vi "Teleop.vi"(10 "Match Info":T1={"Autonomous Elapsed Seconds"=0.0, "TeleOp Elapsed Seconds"=0.0, "Disabled Elapsed Seconds"=0.0, "Visited Autonomous"=FALSE, "Visited TeleOp"=FALSE, "Visited Disabled"=FALSE, "Autonomous Settings"={"Autonomous Style"=enum."Independent", "VI Refnum"=refnum}}, 11 "Call Context":T2) -> ()   [LabVIEW 2014]
doc: "This VI is called for each TeleOp packet received from the DS where the robot is not disabled. It is often used to read from the joysticks and update I/O or to update setpoints for timed control loops. It should complete and return within 20 milliseconds or it may miss DS packets."
uses:
  <vilib>/Rock Robotics/WPI/DriverStation/WPI_DriverStationDerivedRobotMode.ctl
  <vilib>/Rock Robotics/WPI/DriverStation/WPI_DriverStationMatch Info.ctl
  Robot Global Data.vi
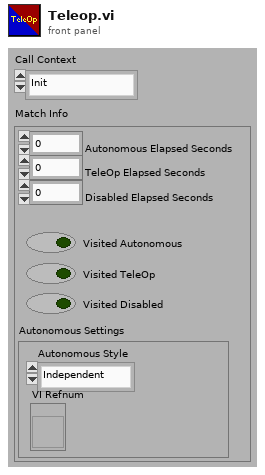
[diagram p1: front panel]
types:
  T1 = typedef "WPI_DriverStationMatch Info.ctl" = cluster{"Autonomous Elapsed Seconds":dbl, "TeleOp Elapsed Seconds":dbl, "Disabled Elapsed Seconds":dbl, "Visited Autonomous":bool, "Visited TeleOp":bool, "Visited Disabled":bool, "Autonomous Settings":cluster{"Autonomous Style":enum16{"Iterative", "Independent"}, "VI Refnum":refnum<vi>}}
  T2 = typedef "WPI_DriverStationDerivedRobotMode.ctl" = enum16{"Init", "Execute", "Stop"}
  T3 = cluster{"axis 3 (throttle)":dbl, "axis 1 (x)":dbl, "axis 2 (y)":dbl}
  T4 = cluster{"Trigger":bool, "Top 1":bool, "Side Trigger":bool, "Top 2":bool, "Top 3":bool, "Top 4":bool, "Bottom 1":bool, "Bottom 2":bool, "Bottom 3":bool, "Bottom 4":bool, "Bottom 5":bool, "Bottom 6":bool}
  T5 = cluster{"axis 1 (x)":dbl, "axis 2 (y)":dbl, "axis 3 (throttle)":dbl, "axis 4":dbl, "axis 5":dbl, "axis 6":dbl}
  T6 = typedef "WPI_AnalogChannelDevRef.ctl" = cluster{"DevStatus":errorcluster, "Analog Module":T7, "Analog Channel":T8}
  T7 = typedef "FPGA_TypedefAnalogModule.ctl" = enum16{"Analog Module 1", "Analog Module 2"}
  T8 = typedef "FPGA_AIChannel.ctl" = enum8{"AI 1", "AI 2", "AI 3", "AI 4", "AI 5", "AI 6", "AI 7", "AI 8", "Invalid"}
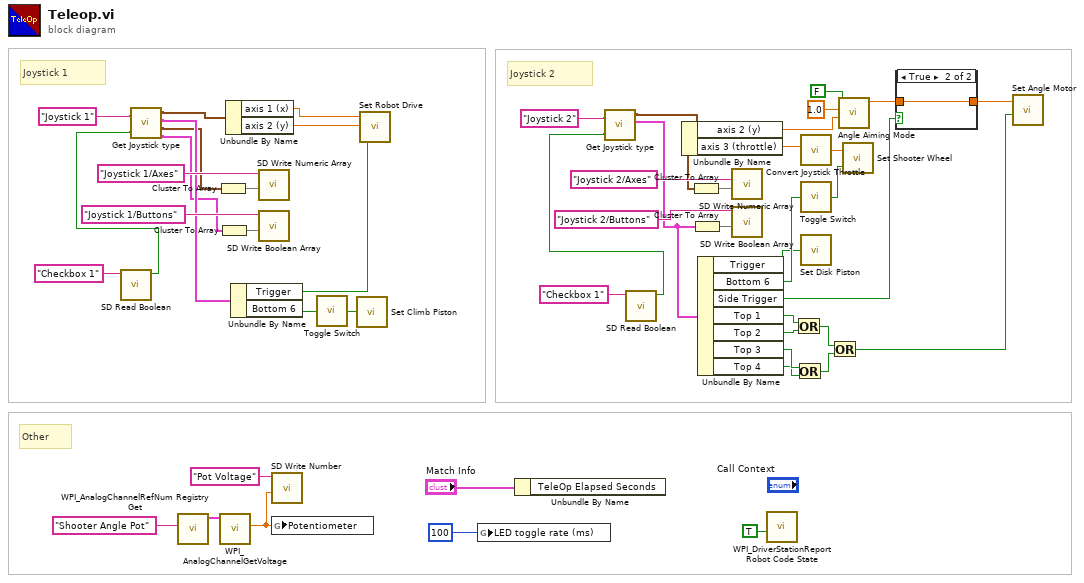
[diagram p0: block diagram]
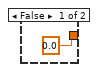
[diagram p2: hidden frame]
diagram:
  # "Other"
  # "Joystick 2"
  # "Joystick 1"
  n1 = call <vilib>:"SD Read Boolean.vi"("Name"="Checkbox 1" ("refnum name")) -> ("Boolean"=w10:bool)  [unwired: 8 in, 2 out]
  n2 = call "Get Joystick type.vi"("refnum name"="Joystick 1", "Pro Joystick"=w10) -> ("Axes"=w8:T3, "Buttons"=w7:T4, "Raw Axes"=w6:T5, "Raw Buttons"=w5:T4)
  n3 = call <vilib>:"WPI_AnalogChannelRefNum Registry Get.vi"("refnum name"="Shooter Angle Pot") -> ("AIDeviceRef"=w28:T6)  [unwired: 9 in, 1 out]
  n4 = Cluster To Array(cluster=w6) -> (array=w45:dbl[])
  n5 = Cluster To Array(cluster=w5) -> (array=w47:bool[])
  n6 = call <vilib>:"WPI_AnalogChannelGetVoltage.vi"("AIDeviceRef"=w28) -> ("Voltage"=w26:dbl)  [unwired: 8 in, 2 out]
  n7 = Unbundle By Name(w8) -> ("axis 1 (x)"=w11:dbl, "axis 2 (y)"=w12:dbl)
  n8 = Unbundle By Name(w7) -> ("Trigger"=w22:bool, "Bottom 6"=w32:bool)
  n9 = call <vilib>:"SD Write Numeric Array.vi"("Numeric Array"=w45, "Name"="Joystick 1/Axes") -> ()  [unwired: 8 in, 2 out]
  n10 = call <vilib>:"SD Write Boolean Array.vi"("Boolean Array"=w47, "Name"="Joystick 1/Buttons") -> ()  [unwired: 8 in, 2 out]
  n11 = call <vilib>:"SD Write Number.vi"("Numeric"=w26, "Name"="Pot Voltage") -> ()  [unwired: 8 in, 2 out]
  n12 = global write "Robot Global Data.vi" "Potentiometer"(w26) -> ()
  n13 = call "Toggle Switch.vi"("Input"=w32) -> ("Output"=w38:bool)
  n14 = call "Set Climb Piston.vi"("Boolean"=w38) -> ()
  n15 = call "Set Robot Drive.vi"("Half Speed"=w22, "Y axis"=w12, "X axis"=w11) -> ()  [unwired: 1 in]
  n16 = global write "Robot Global Data.vi" "LED toggle rate (ms)"(u32 100 ("LED ms toggle rate")) -> ()
  n17 = Unbundle By Name("Match Info") -> ()  [unwired: 1 out]
  n18 = call <vilib>:"SD Read Boolean.vi"("Name"="Checkbox 1" ("refnum name")) -> ("Boolean"=w2:bool)  [unwired: 8 in, 2 out]
  n19 = call "Get Joystick type.vi"("refnum name"="Joystick 2", "Pro Joystick"=w2) -> ("Axes"=w4:T3, "Buttons"=w3:T4)  [unwired: 2 out]
  n20 = Unbundle By Name(w4) -> ("axis 2 (y)"=w35:dbl, "axis 3 (throttle)"=w34:dbl)
  n21 = Cluster To Array(cluster=w4) -> (array=w42:dbl[])
  n22 = Cluster To Array(cluster=w3) -> (array=w40:bool[])
  n23 = Unbundle By Name(w3) -> ("Trigger"=w37:bool, "Bottom 6"=w39:bool, "Side Trigger"=w21:bool, "Top 1"=w16:bool, "Top 2"=w17:bool, "Top 3"=w19:bool, "Top 4"=w18:bool)
  n24 = call <vilib>:"SD Write Numeric Array.vi"("Numeric Array"=w42, "Name"="Joystick 2/Axes") -> ()  [unwired: 8 in, 2 out]
  n25 = call <vilib>:"SD Write Boolean Array.vi"("Boolean Array"=w40, "Name"="Joystick 2/Buttons") -> ()  [unwired: 8 in, 2 out]
  n26 = call <vilib>:"WPI_DriverStationReport Robot Code State.vi"("TeleOp"=TRUE ("Autonomous")) -> ()  [unwired: 10 in, 1 out]
  n27 = Or(x=w16, y=w17) -> (x .or. y?=w20:bool)
  n28 = Or(x=w19, y=w18) -> (x .or. y?=w15:bool)
  n29 = call "Convert Joystick Throttle.vi"("Input"=w34) -> ("Output"=w33:dbl)
  n30 = call "Toggle Switch.vi"("Input"=w39) -> ("Output"=w36:bool)
  n31 = call "Set Disk Piston.vi"("Boolean"=w37) -> ()
  n32 = Or(x=w20, y=w15) -> (x .or. y?=w23:bool)
  n33 = call "Angle Aiming Mode.vi"("Y Axis"=w35, "Motor Scale"=1.0, "Vision Tracking Enable"=FALSE) -> ("Motor Output"=w25:dbl)  [unwired: 8 in]
  n34 = call "Set Shooter Wheel.vi"("Reverse"=w36, "Motor Speed"=w33) -> ()  [unwired: 2 in]
  n35 = case shown="True" w21 {
    tunnel: w25 -> [_ w52]
    tunnel: [0.0 ("Motor Output") w52] -> w24
    frame False {
    }
    frame True {
    }
  }
  n36 = call "Set Angle Motor.vi"("Hold"=w23, "Motor Speed"=w24) -> ()  [unwired: 10 in]
